vi "light_3.vi"() -> ()   [LabVIEW 2010]
panel:
  out "布尔":bool
  in  "枚举":enum16{"无信号", "正常", "不正确"}(ring)
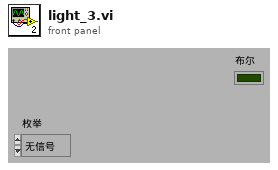
[diagram p1: front panel]
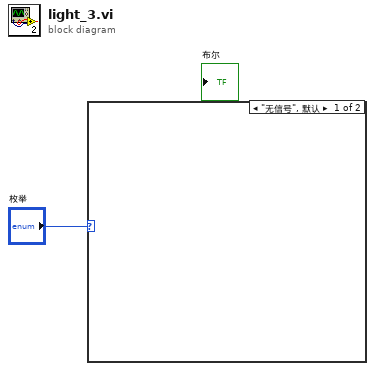
[diagram p0: block diagram]
diagram:
  n1 = case shown="\"无信号\", 默认" "枚举" {
    frame "无信号", Default {
    }
    frame "正常" {
    }
  }
